vi "0-Load Map.vi"(2 "Map Name":T1="Lake Waban", 3 "Image Ref In":T2) -> (0 "Image Descriptor":T3={"Upper-Left Corner Coordinates"={"UTM Zone"=0.0, "Hemisphere"=enum."North", "East"=0.0, "North"=0.0}, "Meters/Pixel"=1.0} {"Upper-Left Corner Coordinates"."North" format="%#_10f"; "Upper-Left Corner Coordinates"."East" format="%#_8f"}, 1 "Image Ref Out":T2)   [LabVIEW 2011]
doc: "Loads a map and its corresponding descriptor text file.\n\n.png will be added to the given Map Name to get the image,\n.txt will be added to get the image descriptor (The image and the descriptor file have the same filename but different extensions)\nfiles will be retrieved from the /locations/ folder."
uses:
  0-Image Descriptor.ctl
  2-Think/2 Typedefs/UTM Location.ctl
  <vilib>/vision/Image Controls.llb/IMAQ Image.ctl
  0 Typedefs/Maps.ctl
panel:
  # ".png will be added to the map name to get the image,\n.txt will be added to get the image descriptor"
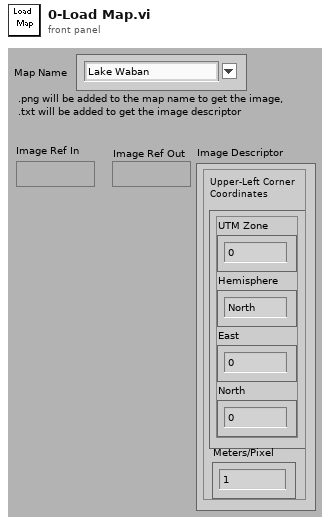
[diagram p1: front panel]
types:
  T1 = typedef "Maps.ctl" = string
  T2 = typedef "IMAQ Image.ctl" = refnum<image>
  T3 = typedef "0-Image Descriptor.ctl" = cluster{"Upper-Left Corner Coordinates":T4, "Meters/Pixel":dbl}
  T4 = typedef "UTM Location.ctl" = cluster{"UTM Zone":dbl, "Hemisphere":enum16{"North", "South"}, "East":dbl, "North":dbl}
  T5 = typedef "Image Type" = u32
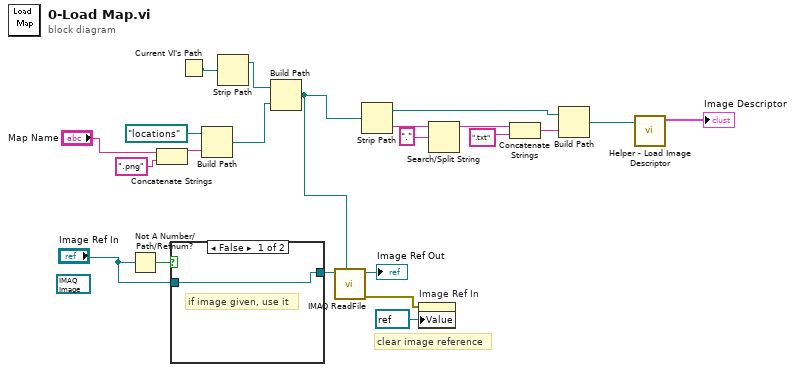
[diagram p0: block diagram]
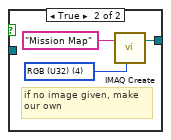
[diagram p2: hidden frame]
diagram:
  (unwired) T2 refnum ("Image Ref In 2")
  # "clear image reference"
  n1 = Not A Number/Path/Refnum?(number/path/refnum="Image Ref In") -> (NaN/Path/Refnum?=w2:bool)
  n2 = Concatenate Strings("Map Name", ".png" ("string")) -> (w9:string)
  n3 = case shown="False" w2 {
    tunnel: [w23 w24] -> w22
    tunnel: "Image Ref In" -> [w23 _]
    frame False {
      # "if image given, use it"
    }
    frame True {
      w25 = T5 4 items=["Grayscale (U8)", "Grayscale (I16)", "Grayscale (SGL)", "Complex (CSG)", "RGB (U32)", "HSL (U32)", "RGB (U64)", "Grayscale (U16)"] ("Image Type")
      # "if no image given, make\nour own"
      n4 = call "IMAQ Create"("Image Name"="Mission Map", "Image Type"=w25) -> ("New Image"=w24:T2)  [unwired: 2 in, 2 out]
    }
  }
  n5 = Current VI's Path() -> (path=w19:path)
  n6 = Build Path(base path=path "locations", name or relative path=w9) -> (appended path=w6:path)
  n7 = Strip Path(path=w19) -> (stripped path=w18:path)  [unwired: 1 out]
  n8 = Build Path(base path=w18, name or relative path=w6) -> (appended path=w10:path)
  n9 = call "IMAQ ReadFile"("File Path"=w10, "Image"=w22) -> ("error out"=w3:errorcluster, "Image Out"=→"Image Ref Out":T2)  [unwired: 3 in, 5 out]
  n10 = Strip Path(path=w10) -> (stripped path=w13:path, name=w14:string)
  n11 = property on="Image Ref In" class="IMAQImage (strict)"(error in=w3, "Value"=refnum<image> refnum) -> ()  [unwired: 1 in, 2 out]
  n12 = Search/Split String(string=w14, search string/char (-)=".") -> (substring before match=w15:string)  [unwired: 3 out]
  n13 = Concatenate Strings(w15, ".txt" ("string")) -> (w17:string)
  n14 = Build Path(base path=w13, name or relative path=w17) -> (appended path=w12:path)
  n15 = call "Helper - Load Image Descriptor.vi"("Image Descriptor File Path"=w12) -> ("Image Descriptor Typedef out"=→"Image Descriptor":T3)  [unwired: 10 in]
